vi "Parse SNMP Packet Header.vi"(8 "error in (no error)":errorcluster, 11 "SNMP Packet":u8[](array[numeric]) format="%.0x") -> (0 "error out":errorcluster, 1 "Req ID":i32, 3 "SNMP Packet Out":u8[](array[numeric]) format="%.0x", 4 "Error Index":i32, 5 "Community String":string, 6 "Error Status":i32, 7 "SNMP version":i32)   [LabVIEW 2017]
doc: "This VI is used to parse the SNMP packet header into its components parts."
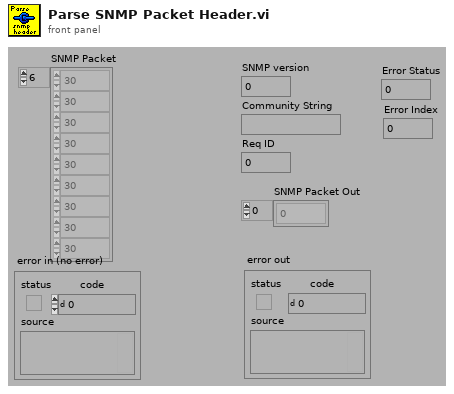
[diagram p1: front panel]
types:
  T1 = cluster{"Numeric":u32, "Octet String":string, "Byte Array":u8[]}
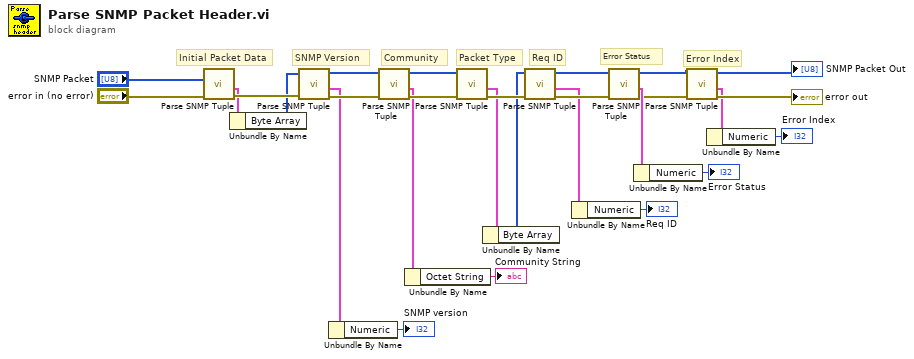
[diagram p0: block diagram]
diagram:
  # "Error Index"
  # "Error Status"
  # "Packet Type"
  # "Req ID"
  # "Community"
  # "SNMP Version"
  # "Initial Packet Data"
  n1 = call "Parse SNMP Tuple.vi"("error in (no error)"="error in (no error)", "SNMP Packet In"="SNMP Packet") -> ("error out"=w25:errorcluster, "Data Out"=w12:T1)  [unwired: 8 out]
  n2 = Unbundle By Name(w12) -> ("Byte Array"=w11:u8[])
  n3 = call "Parse SNMP Tuple.vi"("error in (no error)"=w25, "SNMP Packet In"=w11) -> ("error out"=w24:errorcluster, "Data Out"=w19:T1, "SNMP Packet Out"=w27:u8[])  [unwired: 7 out]
  n4 = Unbundle By Name(w19) -> ("Numeric"=→"SNMP version":u32)
  n5 = call "Parse SNMP Tuple.vi"("error in (no error)"=w24, "SNMP Packet In"=w27) -> ("error out"=w23:errorcluster, "Data Out"=w17:T1, "SNMP Packet Out"=w26:u8[])  [unwired: 7 out]
  n6 = Unbundle By Name(w17) -> ("Octet String"=→"Community String":string)
  n7 = call "Parse SNMP Tuple.vi"("error in (no error)"=w23, "SNMP Packet In"=w26) -> ("error out"=w22:errorcluster, "Data Out"=w15:T1)  [unwired: 8 out]
  n8 = Unbundle By Name(w15) -> ("Byte Array"=w10:u8[])
  n9 = call "Parse SNMP Tuple.vi"("error in (no error)"=w22, "SNMP Packet In"=w10) -> ("error out"=w20:errorcluster, "Data Out"=w14:T1, "SNMP Packet Out"=w21:u8[])  [unwired: 7 out]
  n10 = Unbundle By Name(w14) -> ("Numeric"=→"Req ID":u32)
  n11 = call "Parse SNMP Tuple.vi"("error in (no error)"=w20, "SNMP Packet In"=w21) -> ("error out"=w6:errorcluster, "Data Out"=w8:T1, "SNMP Packet Out"=w5:u8[])  [unwired: 7 out]
  n12 = Unbundle By Name(w8) -> ("Numeric"=→"Error Status":u32)
  n13 = call "Parse SNMP Tuple.vi"("error in (no error)"=w6, "SNMP Packet In"=w5) -> ("error out"=→"error out":errorcluster, "Data Out"=w2:T1, "SNMP Packet Out"=→"SNMP Packet Out":u8[])  [unwired: 7 out]
  n14 = Unbundle By Name(w2) -> ("Numeric"=→"Error Index":u32)
